vi "rszvl Configure SAN Reference Level.vi"(8 "error in (no error)":errorcluster, 9 "Reference Level (-20.0)":dbl=-20.0 format="%^.3e", 11 "VISA resource name":refnum<visa-resource-name>) -> (0 "error out":errorcluster, 3 "VISA resource name out":refnum<visa-resource-name>)   [LabVIEW 2014]
doc: "This VI configures the reference level\n\nAttribute(s):\nRSZVL_ATTR_REFERENCE_LEVEL\n\nRemote-control command(s):\nDISPlay[:WINDow<1|2>]:TRACe<1…3>:Y[:SCALe]:RLEVel"
uses:
  Instance           1 43Saved   rszvl Configure SAN Reference Level .vi
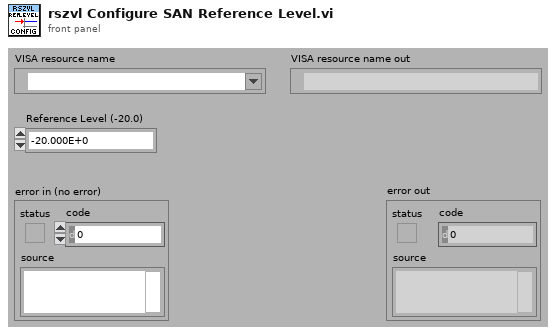
[diagram p1: front panel]
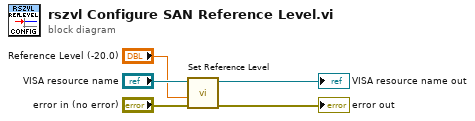
[diagram p0: block diagram]
diagram:
  n1 = call "Set Reference Level"("error in (no error)"="error in (no error)", "Reference Level (0.0)"="Reference Level (-20.0)", "instrument handle"="VISA resource name") -> ("error out"=→"error out":errorcluster, "instrument handle out"=→"VISA resource name out":refnum<visa-resource-name>)  [unwired: 7 in]
